vi "read_params.vi"(8 "error in (no error)":errorcluster, 11 "FastICA in":refnum<class "FastICA.lvclass">) -> (0 "error out":errorcluster, 2 "params":T1={"n_components"={"n_components_type"="None", "n_components_int"=0.0}, "algorithm"="parallel", "whiten"=TRUE, "fun"="logcosh", "max_iter"=200.0, "tol"=0.0001, "w_init"={"w_init_type"="None", "w_init_list"=[]}, "random_state"=0.0}, 3 "FastICA out":refnum<class "FastICA.lvclass">)   [LabVIEW 2020, in "FastICA.lvclass"]
uses:
  FastICA.lvclass
  Controls/fast_ica_params.ctl
  FastICA.lvclass/FastICA.ctl
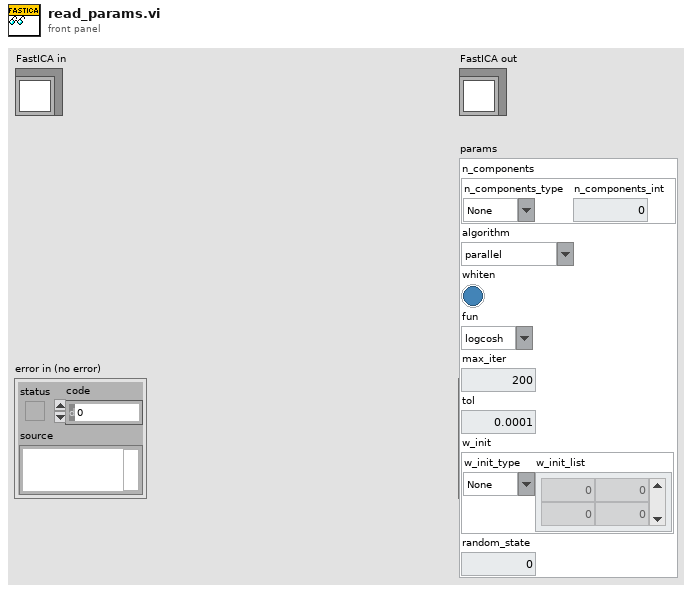
[diagram p1: front panel]
types:
  T1 = typedef "fast_ica_params.ctl" = cluster{"n_components":cluster{"n_components_type":string, "n_components_int":dbl}, "algorithm":string, "whiten":bool, "fun":string, "max_iter":dbl, "tol":dbl, "w_init":cluster{"w_init_type":string, "w_init_list":dbl[][]}, "random_state":dbl}
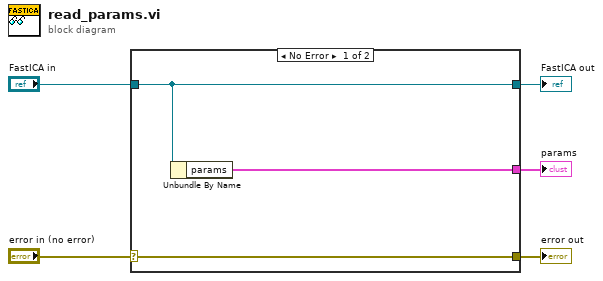
[diagram p0: block diagram]
diagram:
  n1 = case shown="No Error" "error in (no error)" {
    selector: "error in (no error)" -> [w8 w9]
    tunnel: [w8 w9] -> w4
    tunnel: [w7 w10] -> w2
    tunnel: "FastICA in" -> [w7 w10]
    tunnel: [w6 _] -> w1
    frame No Error {
      n2 = Unbundle By Name(w7) -> ("params"=w6:T1)
    }
    frame Error {
    }
  }
  "error out" <- w4
  "FastICA out" <- w2
  "params" <- w1
